vi "ЛР6 - 3 варик.vi"() -> ()   [LabVIEW 2012]
uses:
  <vilib>/Analysis/3filter.llb/Filter Passband Type.ctl
  <vilib>/Analysis/3filter.llb/Inverse Chebyshev Filter (DBL).vi
  <vilib>/Analysis/2dsp.llb/Real FFT.vi
  <vilib>/Analysis/NI_AALBase.lvlib
  <vilib>/Analysis/NI_AALPro.lvlib
panel:
  out "Phase":cluster{"y":dbl, dbl, dbl[]}(graph)
  out "Amplitude":cluster{"y":dbl, dbl, dbl[]}(graph)
  in  "Scale Phase":bool
  in  "Scale Amplitude":bool
  in  "Chebyshev Filter":T2={"filter type"=enum."Lowpass", "order"=2, "ripple(dB)"=0.1, "sampling freq: fs"=1.0, "high cutoff freq: fh"=0.45000000000000007, "low cutoff freq: fl"=0.125} {"low cutoff freq: fl" scale=0.0..1.0; "high cutoff freq: fh" scale=0.0..1.0; "sampling freq: fs" scale=0.0..10.0; "ripple(dB)" format="%0.2f"}
  # "Abs"
  # "dB"
  # "Road"
  # "Grad"
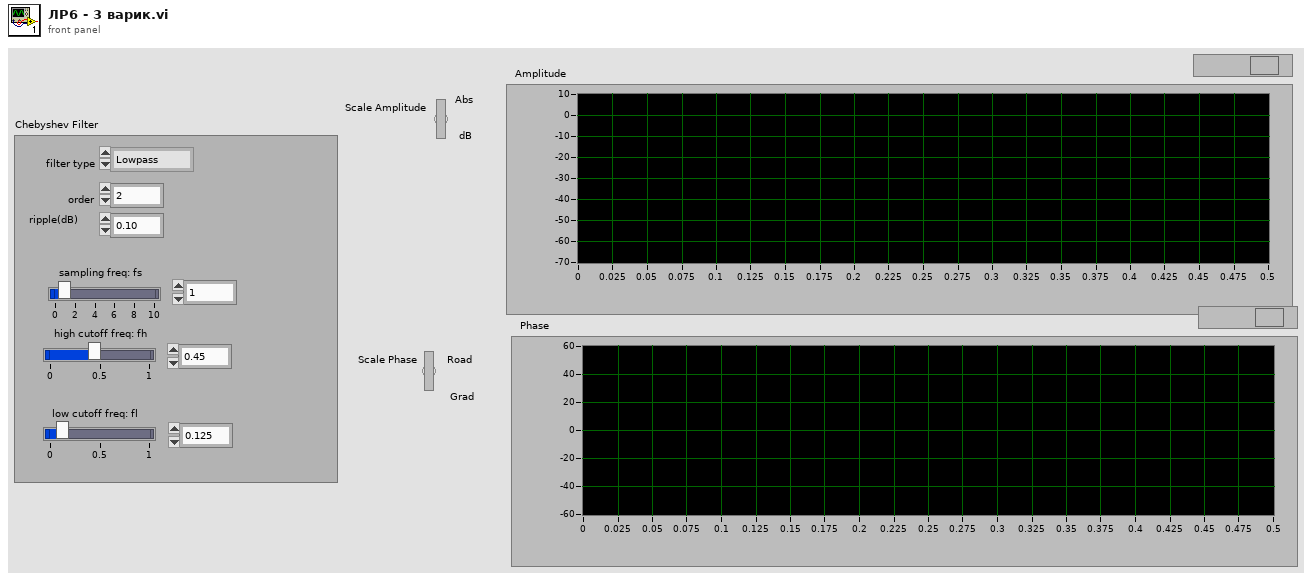
[diagram p1: front panel]
types:
  T1 = typedef "NI_AALBase.lvlib/Filter Passband Type.ctl" = enum32{"Lowpass", "Highpass", "Bandpass", "Bandstop"}
  T2 = cluster{"filter type":T1, "order":i32, "ripple(dB)":dbl, "sampling freq: fs":dbl, "high cutoff freq: fh":dbl, "low cutoff freq: fl":dbl}
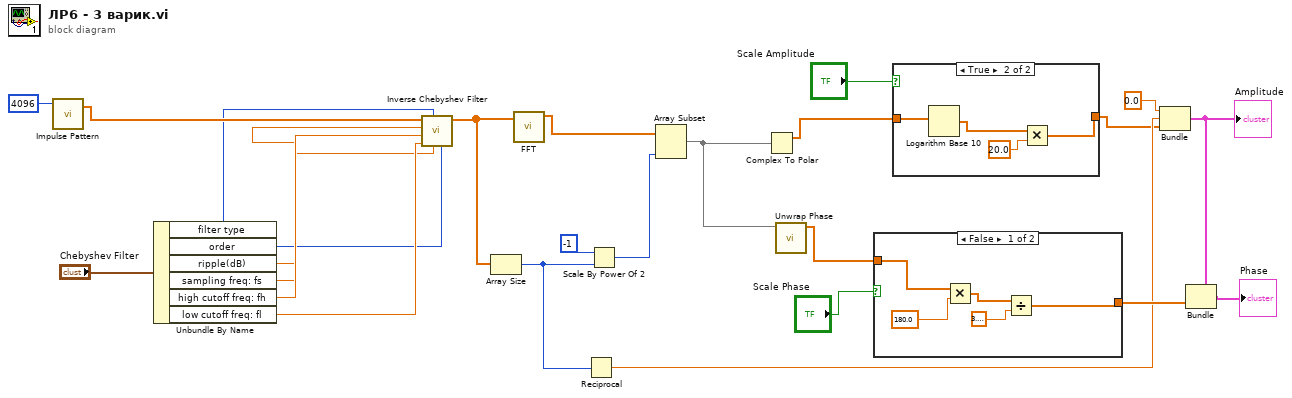
[diagram p0: block diagram]
diagram:
  n1 = call <vilib>:"Impulse Pattern.vi"("samples"=4096) -> ("Impulse Pattern"=w24:dbl[])  [unwired: 2 in, 1 out]
  n2 = Unbundle By Name("Chebyshev Filter") -> ("filter type"=w17:T1, "order"=w18:i32, "ripple(dB)"=w19:dbl, "sampling freq: fs"=w20:dbl, "high cutoff freq: fh"=w21:dbl, "low cutoff freq: fl"=w22:dbl)
  n3 = call-poly <vilib>:"Inverse Chebyshev Filter.vi"("order"=w18, "attenuation (dB)"=w19, "filter type"=w17, "low cutoff freq: fl"=w22, "high cutoff freq: fh"=w21, "sampling freq: fs"=w20, "X"=w24) -> ("Filtered X"=w16:dbl[])  [unwired: 3 in, 1 out]
  n4 = Array Size(array=w16) -> (size(s)=w15:i32)
  n5 = call-poly <vilib>:"FFT.vi"("X"=w16) -> ("FFT {X}"=w13:cdb[])  [unwired: 9 in, 1 out]
  n6 = Reciprocal(x=w15) -> (1/x=w7:dbl)
  n7 = Scale By Power Of 2(n=i16 -1, x=w15) -> (x*2^n=w12:i32)
  n8 = Array Subset(array=w13, length=w12) -> (w11:cdb[])  [unwired: 1 in]
  n9 = Complex To Polar(r * e^(i*theta)=w11) -> (r=w10:dbl[])  [unwired: 1 out]
  n10 = call <vilib>:"Unwrap Phase.vi"("Phase"=w11) -> ("Unwrapped Phase"=w9:dbl[])  [unwired: 9 in, 1 out]
  n11 = case shown="False" "Scale Phase" {
    tunnel: w9 -> [w30 w31]
    tunnel: [w27 w31] -> w8
    frame False {
      n12 = Multiply(x=w30, y=180.0) -> (x*y=w29:dbl[])
      n13 = Divide(x=w29, y=3.141592653589793) -> (x/y=w27:dbl[])
    }
    frame True {
    }
  }
  n14 = case shown="True" "Scale Amplitude" {
    tunnel: w10 -> [w32 w35]
    tunnel: [w32 w33] -> w6
    frame False {
    }
    frame True {
      n15 = Logarithm Base 10(1:w35) -> (0:w34:dbl[])
      n16 = Multiply(x=w34, y=20.0) -> (x*y=w33:dbl[])
    }
  }
  n17 = Bundle "Bundle"("y"=0.0, w7, w6) -> (w4:cluster{"y":dbl, dbl, dbl[]})  [unwired: 1 in]
  "Amplitude" <- w4
  n18 = Bundle "Bundle"(cluster=w4, w8) -> (→"Phase":cluster{"y":dbl, dbl, dbl[]})  [unwired: 2 in]
